vi "INIfileOperator.vi"(7 "Command":enum16{"Write", "Read", "Write Default Path"}(ring), 8 "error in (no error)":errorcluster, 11 "Last Path":path) -> (0 "error out":errorcluster, 3 "Last Path output":path)   [LabVIEW 2017]
uses:
  <vilib>/Utility/config.llb/NI_LVConfig.lvlib
  <vilib>/Utility/config.llb/Write Key (Path).vi
  <vilib>/Utility/config.llb/Read Key (Path).vi
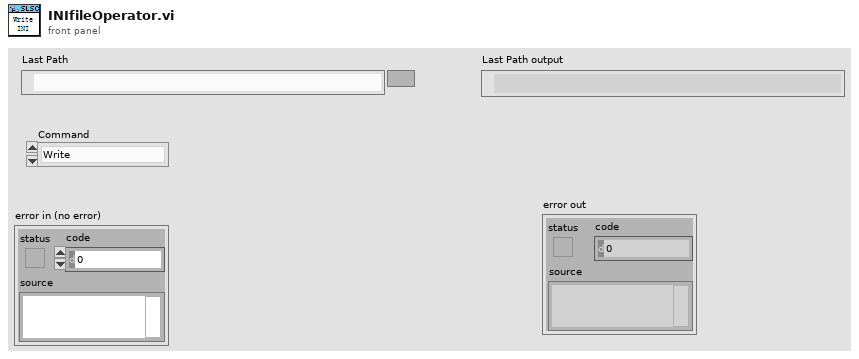
[diagram p1: front panel]
types:
  T1 = typedef "NI_LVConfig.lvlib/Config Data RefNum.ctl" = refnum<k1>
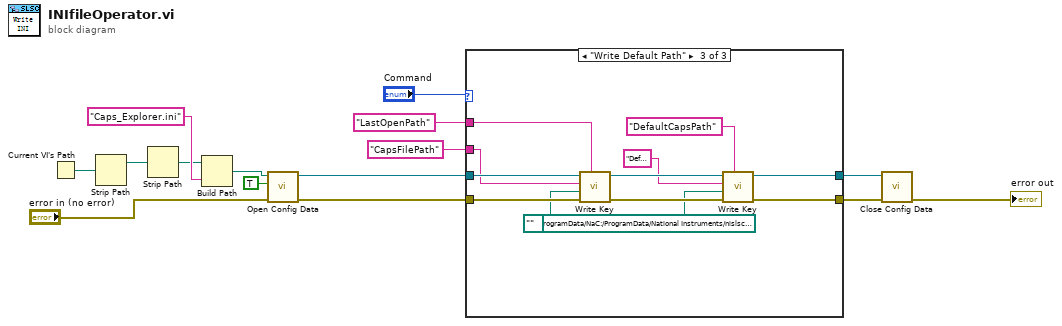
[diagram p0: block diagram]
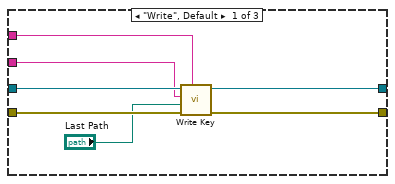
[diagram p2: hidden frame]
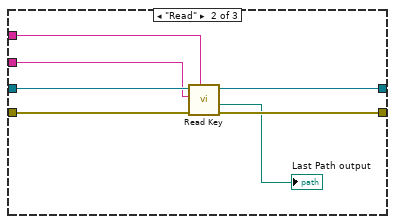
[diagram p3: hidden frame]
diagram:
  n1 = Current VI's Path() -> (path=w15:path)
  n2 = Strip Path(path=w15) -> (stripped path=w14:path)  [unwired: 1 out]
  n3 = Strip Path(path=w14) -> (stripped path=w1:path)  [unwired: 1 out]
  n4 = Build Path(base path=w1, name or relative path="Caps_Explorer.ini") -> (appended path=w12:path)
  n5 = call <vilib>:"Open Config Data.vi"("error in (no error)"="error in (no error)", "create file if necessary (T)"=TRUE, "configuration file path"=w12) -> ("error out"=w9:errorcluster, "refnum"=w8:T1)  [unwired: 6 in, 1 out]
  n6 = case shown="\"Write Default Path\"" "Command" {
    tunnel: w9 -> [w22 w28 w36]
    tunnel: w8 -> [w21 w29 w37]
    tunnel: [w19 w26 w40] -> w5
    tunnel: [w18 w27 w41] -> w6
    tunnel: "LastOpenPath" ("section") -> [w17 w25 w35]
    tunnel: "CapsFilePath" ("key") -> [w16 w24 w34]
    frame "Write", Default {
      n7 = call-poly <vilib>:"Write Key.vi"("section"=w17, "error in (no error)"=w22, "value"="Last Path", "key"=w16, "refnum"=w21) -> ("error out"=w19:errorcluster, "refnum out"=w18:T1)  [unwired: 4 in, 1 out]
    }
    frame "Read" {
      n8 = call-poly <vilib>:"Read Key.vi"("section"=w25, "error in (no error)"=w28, "key"=w24, "refnum"=w29) -> ("error out"=w26:errorcluster, "value"=→"Last Path output":path, "refnum out"=w27:T1)  [unwired: 4 in, 1 out]
    }
    frame "Write Default Path" {
      n9 = call-poly <vilib>:"Write Key.vi"("section"=w35, "error in (no error)"=w36, "value"=path "", "key"=w34, "refnum"=w37) -> ("error out"=w38:errorcluster, "refnum out"=w39:T1)  [unwired: 4 in, 1 out]
      n10 = call-poly <vilib>:"Write Key.vi"("section"="DefaultCapsPath", "error in (no error)"=w38, "value"=path "C:/ProgramData/NaC:/ProgramData/National Instruments/nislsc/capabilities", "key"="DefaultCapsFilePath", "refnum"=w39) -> ("error out"=w40:errorcluster, "refnum out"=w41:T1)  [unwired: 4 in, 1 out]
    }
  }
  n11 = call <vilib>:"Close Config Data.vi"("error in (no error)"=w5, "refnum"=w6) -> ("error out"=→"error out":errorcluster)  [unwired: 8 in, 1 out]
